vi "Plugin.Tx.vi"(8 "error in (no error)":errorcluster, 10 "Transfer Group":refnum<class "DSF.Engine.Transfer Group.lvclass">, 11 "UDP Plugin in":refnum<class "UDP Plugin.lvclass">) -> (0 "error out":errorcluster, 3 "UDP Plugin out":refnum<class "UDP Plugin.lvclass">)   [LabVIEW 2016, in "UDP Plugin.lvclass"]
uses:
  UDP Plugin.lvclass
  Source/Engine/Classes/Transfer/DSF.Engine.Transfer Group.lvclass
  Plugin.lvclass
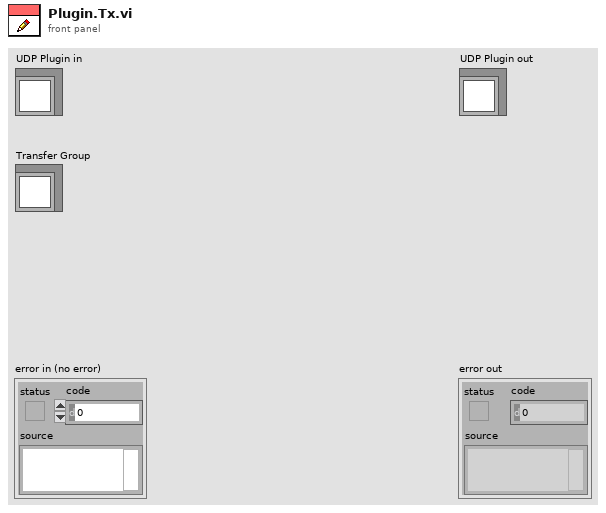
[diagram p1: front panel]
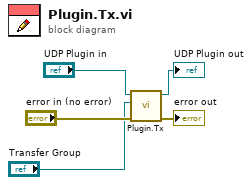
[diagram p0: block diagram]
diagram:
  n1 = call-parent "Plugin.Tx.vi"("error in (no error)"="error in (no error)", "Transfer Group"="Transfer Group", "Plugin in"="UDP Plugin in") -> ("error out"=→"error out":errorcluster, "Plugin out"=→"UDP Plugin out":refnum<class "UDP Plugin.lvclass">)  [unwired: 7 in]
